vi "Screen Size.vi"() -> ()   [LabVIEW 2016]
uses:
  <vilib>/Utility/miscctls.llb/LVRectTypeDef.ctl
panel:
  out "Win Height":i16
  out "Win Width":i16
  out "Panel Height":i16
  out "Panel Width":i16
  in  "Set to TVAC screen":bool
  out "Front Panel Window:Window Bounds":T1
  out "Front Panel Window:Panel Bounds":T1
  in  "stop":bool
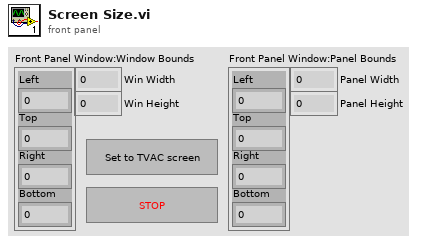
[diagram p1: front panel]
types:
  T1 = typedef "LVRectTypeDef.ctl" = cluster{"Left":i16, "Top":i16, "Right":i16, "Bottom":i16}
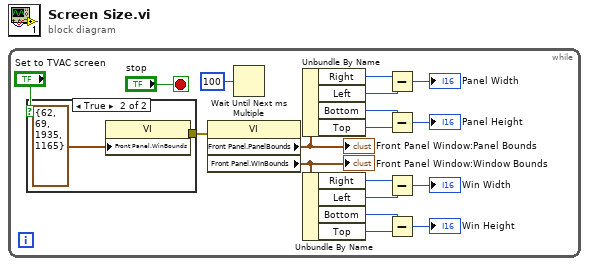
[diagram p0: block diagram]
diagram:
  n1 = while {
    stop <- "stop" stop-if-true
    n2 = case shown="True" "Set to TVAC screen" {
      tunnel: [_ w20] -> w16
      frame False {
      }
      frame True {
        n3 = property on="Property Node" class="VI"("Front Panel.WinBounds"=T1 {"Left"=62, "Top"=69, "Right"=1935, "Bottom"=1165} ("Front Panel Window:Window Bounds 2")) -> (error out=w20:errorcluster)  [unwired: 2 in, 1 out]
      }
    }
    n4 = property on="Property Node" class="VI"(error in=w16) -> ("Front Panel.PanelBounds"=w14:T1, "Front Panel.WinBounds"=w13:T1)  [unwired: 1 in, 2 out]
    "Front Panel Window:Panel Bounds" <- w14
    "Front Panel Window:Window Bounds" <- w13
    n5 = Wait Until Next ms Multiple(millisecond multiple=u32 100) -> ()  [unwired: 1 out]
    n6 = Unbundle By Name(w14) -> ("Right"=w12:i16, "Left"=w11:i16, "Bottom"=w10:i16, "Top"=w9:i16)
    n7 = Unbundle By Name(w13) -> ("Right"=w8:i16, "Left"=w7:i16, "Bottom"=w6:i16, "Top"=w5:i16)
    n8 = Subtract(x=w12, y=w11) -> (x-y=→"Panel Width":i16)
    n9 = Subtract(x=w10, y=w9) -> (x-y=→"Panel Height":i16)
    n10 = Subtract(x=w8, y=w7) -> (x-y=→"Win Width":i16)
    n11 = Subtract(x=w6, y=w5) -> (x-y=→"Win Height":i16)
  }
